vi "Editor Context.vi"(10 "Close (F)":bool, 11 "Context":T1) -> (2 "error out":errorcluster, 3 "Editor Context":refnum<vi>)   [LabVIEW 2020, in "Conditum-Tools.lvlib"]
uses:
  Conditum-Tools.lvlib
  Context.ctl
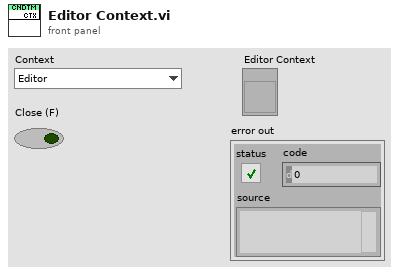
[diagram p1: front panel]
types:
  T1 = typedef "Conditum-Tools.lvlib/Context.ctl" = enum16{"Editor", "Entity"}
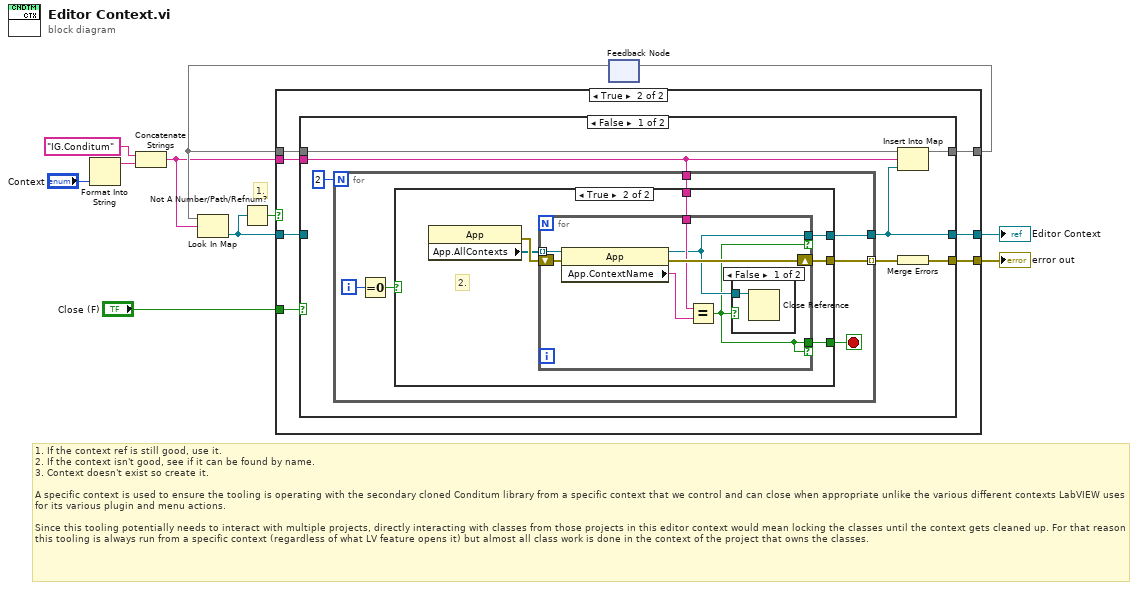
[diagram p0: block diagram]
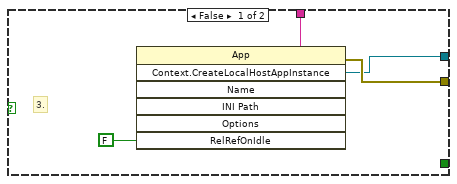
[diagram p3: hidden frame]
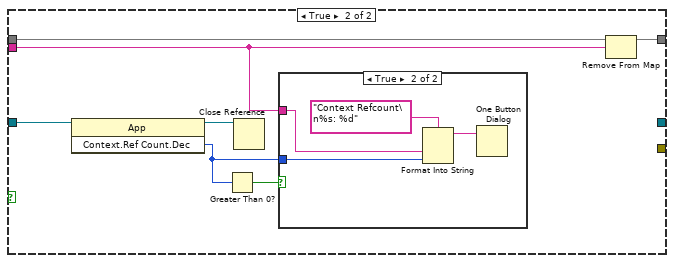
[diagram p5: hidden frame]
diagram:
  # "1."
  # "1. If the context ref is still good, use it.\n2. If the context isn't good, see if it can be found by name.\n3. Context doesn't exist so create it.\n\nA specific context is used to ensure the tooling is operating with the secondary cloned Conditum library from a specific context that we control and can close when appropriate unlike the various different contexts LabVIEW uses for its various plugin and menu actions.\n\nSince this tooling potentially needs to interact with multiple projects, directly interacting with classes from those projects in this editor context would mean locking the classes until the context gets cleaned up. For that reason this tooling is always run from a specific context (regardless of what LV feature opens it) but almost all class work is done in the context of the project that owns the classes."
  n1 = Format Into String("Context") -> (resulting string=w5:string)  [unwired: 3 in, 1 out]
  n2 = Concatenate Strings("IG.Conditum" ("string"), w5) -> (w3:string)
  n3 = feedback #1() -> (w7:map{string, refnum<vi>})  [unwired: 1 in]
  n4 = Look In Map(map=w7, key=w3) -> (value=w9:refnum<vi>)  [unwired: 1 in, 1 out]
  n5 = Not A Number/Path/Refnum?(number/path/refnum=w9) -> (NaN/Path/Refnum?=w8:bool)
  n6 = case shown="True" w8 {
    tunnel: w3 -> [_ w17]
    tunnel: [w13 w18] -> w10
    tunnel: [_ w20] -> w11
    tunnel: w9 -> [w13 w14]
    tunnel: w7 -> [w12 w19]
    tunnel: [w12 w16] -> w6
    tunnel: "Close (F)" -> [_ w15]
    frame False {
    }
    frame True {
      n7 = case shown="False" w15 {
        tunnel: [w25 _] -> w20
        tunnel: w19 -> [w24 w58]
        tunnel: [w23 _] -> w18
        tunnel: w17 -> [w22 w52]
        tunnel: [w21 w57] -> w16
        tunnel: w14 -> [_ w56]
        frame False {
          n8 = for {
            N: 2 -> [_]
            tunnel: w22 -> [w31]
            tunnel: [w29] -> w23
            tunnel: [w28] -> w26 mode=indexing
            i -> [w33]
            stop <- w30 stop-if-true
            n9 = Equal To 0?(x=w33) -> (x = 0?=w32:bool)
            n10 = case shown="True" w32 {
              tunnel: w31 -> [w35 w38]
              tunnel: [_ w41] -> w30
              tunnel: [w36 w39] -> w29
              tunnel: [w37 w40] -> w28
              frame False {
                # "3."
                n11 = invoke class="App" method="Context.CreateLocalHostAppInstance"("Name"=w35, "RelRefOnIdle"=FALSE ("Release Ref on Idle (T)")) -> (error out=w37:errorcluster, "Create Context"=w36:refnum<vi>)  [unwired: 5 in, 5 out]
              }
              frame True {
                # "2."
                n12 = property class="App"() -> (error out=w43:errorcluster, "App.AllContexts"=w42:refnum<vi>[])  [unwired: 2 in, 1 out]
                n13 = for {
                  tunnel: w38 -> [w48]
                  tunnel: w42 -> [w49] mode=indexing
                  tunnel: [w46] -> w39 if=w45
                  tunnel: [w45] -> w41 if=w45
                  shift-right: [w50] -> w40
                  shift-left: w43 -> [w44]
                  n14 = property class="App"(reference=w49, error in=w44) -> (reference out=w46:refnum<vi>, error out=w50:errorcluster, "App.ContextName"=w47:string)
                  n15 = Equal?(x=w48, y=w47) -> (x = y?=w45:bool)
                  n16 = case shown="False" w45 {
                    tunnel: w46 -> [w51 _]
                    frame False {
                      n17 = Close Reference(reference=w51) -> ()  [unwired: 1 in, 1 out]
                    }
                    frame True {
                    }
                  }
                }
              }
            }
          }
          n18 = Insert Into Map(map in=w24, key=w22, value=w23) -> (map out=w21:map{string, refnum<vi>})  [unwired: 2 out]
          n19 = Merge Errors(w26) -> (w25:errorcluster)
        }
        frame True {
          n20 = invoke class="App" method="Context.Ref Count.Dec"(reference=w56) -> (reference out=w55:refnum<vi>, "Context.Ref Count.Dec"=w53:i32)  [unwired: 2 in, 1 out]
          n21 = Greater Than 0?(x=w53) -> (x > 0?=w54:bool)
          n22 = Close Reference(reference=w55) -> ()  [unwired: 1 in, 1 out]
          n23 = case shown="True" w54 {
            tunnel: w53 -> [_ w60]
            tunnel: w52 -> [_ w61]
            frame False {
            }
            frame True {
              n24 = Format Into String(format string="Context Refcount\n%s: %d", w61, w60) -> (resulting string=w59:string)  [unwired: 2 in, 1 out]
              n25 = One Button Dialog(message=w59) -> ()  [unwired: 1 in, 1 out]
            }
          }
          n26 = Remove From Map(10:w52, 11:w58) -> (3:w57:map{string, refnum<vi>})  [unwired: 2 out]
        }
      }
    }
  }
  "Editor Context" <- w10
  "error out" <- w11
  n27 = feedback-in #1(w6) -> ()
